vi "Construct - Input (Binary).vi"(4 "extension":string, 5 "N Day Buffer":u32, 6 "file name format":string="Log %<%Y-%m-%d %H%M%S>T", 7 "Max File Size (MB)":dbl=512.0, 8 "Layout Type":refnum<class "Layout.lvclass">, 9 "Name":string, 10 "Level":T1=enum."DEBUG", 11 "log location":path) -> (0 "Error Out":errorcluster, 3 "Text File - Binary":refnum<class "Text File - Binary.lvclass">)   [LabVIEW 2019, in "TSC Event Logger.lvlib" / "Text File - Binary.lvclass"]
uses:
  Text File - Binary.lvclass
  C:/Development/Reuse-libraries/Event Logger/Log Sinks/Text File/Text File.lvclass
  Log/Event Level.ctl
  Layouts/Layout.lvclass
  Text File/Text File.lvclass
  TSC Event Logger.lvlib
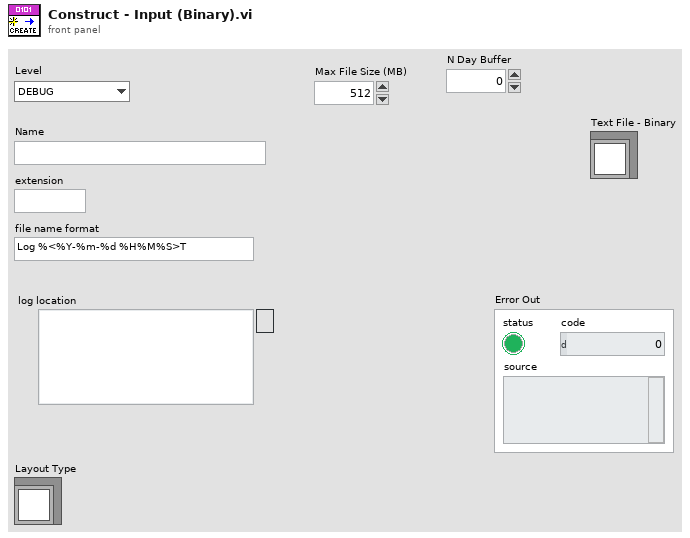
[diagram p1: front panel]
types:
  T1 = typedef "TSC Event Logger.lvlib/Event Level.ctl" = enum16{"OFF", "TRACE", "DEBUG", "INFO", "WARN", "ERROR", "FATAL"}
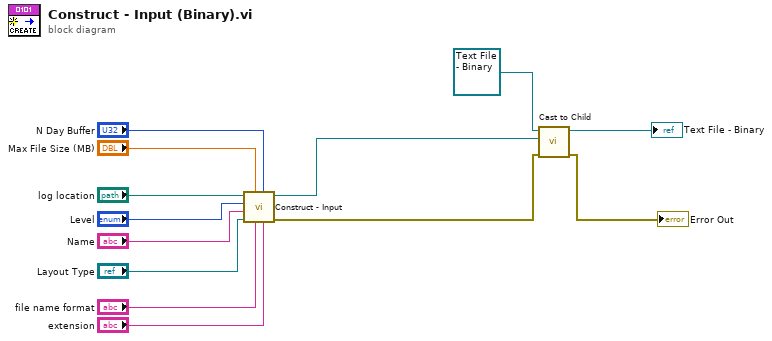
[diagram p0: block diagram]
diagram:
  n1 = call "Construct - Input.vi"("extension"="extension", "N Day Buffer"="N Day Buffer", "file name format"="file name format", "Max File Size (MB)"="Max File Size (MB)", "Layout Type"="Layout Type", "Name"="Name", "Level"="Level", "log location"="log location") -> ("Error Out"=w3:errorcluster, "Text File"=w4:refnum<class "Text File.lvclass">)  [unwired: 2 in]
  n2 = call "Cast to Child.vi"("error in (no error)"=w3, "Parent"=w4, "Child in"=refnum<class "Text File - Binary.lvclass"> refnum ("TSC Event Logger.lvlib:Text File - Binary.lvclass")) -> ("error out"=→"Error Out":errorcluster, "Child Out"=→"Text File - Binary":refnum<class "Text File - Binary.lvclass">)  [unwired: 7 in]
